vi "pump rpm all tubing.vi"(0 "Pump":T1 {"0 to 1" format="%.2f"; "flow rate" format="%.2f"}, 1 "pump ID":u8) -> (2 "pump U8":u8, 3 "pump speed (rpm)":dbl format="%.2f", 4 "command chars":string[](array[string]), 5 "in range":bool)   [LabVIEW 2012]
uses:
  Peristaltic/Pump w direction.ctl
  mini peristaltic pump.ctl
  Pump Direction.ctl
  3-stop colors and numbers.ctl
  calibration commands.ctl
panel:
  out "x+y":dbl
  in  "mL per rev":sgl[](array[numeric])=[0.001518497, 0.003209591, 0.005497798, 0.012406906, 0.016451517, 0.021816157, 0.026944764, 0.03351825, 0.04617598, 0.061704744, 0.069453366, 0.0789204, 0.088816434, 0.09612975, 0.10822253, 0.12075485, 0.14027181, 0.15709075, 0.17954482, 0.19715126, 0.2149444, 0.252498, 0.29306096, 0.3351765, 0.37380016, 0.42250744, 0.06, 0.21, 1.7, 0.8, 2.8, 3.8] format="%.7f"
  in  "IDs":sgl[](array[numeric])=[0.13, 0.19, 0.25, 0.38, 0.44, 0.51, 0.57, 0.64, 0.76, 0.89, 0.95, 1.02, 1.09, 1.14, 1.22, 1.3, 1.42, 1.52, 1.65, 1.75, 1.85, 2.06, 2.29, 2.54, 2.79, 3.17, 0.79375, 1.5875, 4.8, 3.175, 6.35, 7.9375] format="%.3f"
  # "orange-black\norange-red\norange-blue\norange-green\ngreen-yellow\norange-yellow\nwhite-yellow\norange-white\nblack-black\norange-orange\nwhite-black\nwhite-white\nwhite-red\nred-red\nred-grey\ngrey-grey\nyellow-yellow\nyellow-blue\nblue-blue\nblue-green\ngreen-green\npurple-purple\npurple-black\npurple-orange\npurple-white\nblack-white\n13\n14\n15\n16\n17\n18"
  # "13"
  # "14"
  # "15"
  # "16"
  # "17"
  # "18"
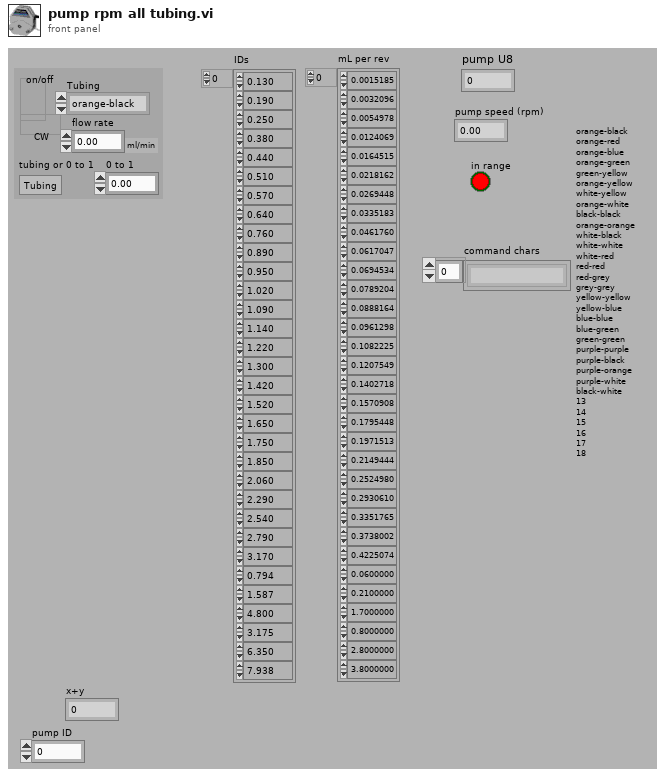
[diagram p1: front panel]
types:
  T1 = typedef "Pump w direction.ctl" = cluster{"on/off":T2, "Direction":T3, "flow rate":dbl[unit], "Tubing":T4, "tubing or 0 to 1":bool, "0 to 1":dbl}
  T2 = typedef "mini peristaltic pump.ctl" = bool
  T3 = typedef "Pump Direction.ctl" = bool
  T4 = typedef "3-stop colors and numbers.ctl" = enum16{"orange-black", "orange-red", "orange-blue", "orange-green", "green-yellow", "orange-yellow", "white-yellow", "orange-white", "black-black", "orange-orange", "white-black", "white-white", "white-red", "red-red", "red-grey", "grey-grey", "yellow-yellow", "yellow-blue", "blue-blue", "blue-green", "green-green", "purple-purple", "purple-black", "purple-orange", "purple-white", "black-white", "13", "14", "15", "16", "17", "18"}
  T5 = typedef "calibration commands.ctl" = enum16{"Get ini Path", "Save default values", "Save new calibration", "Read calibration", "Apply calibration", "Read STAMP mb", "Write STAMP mb"}
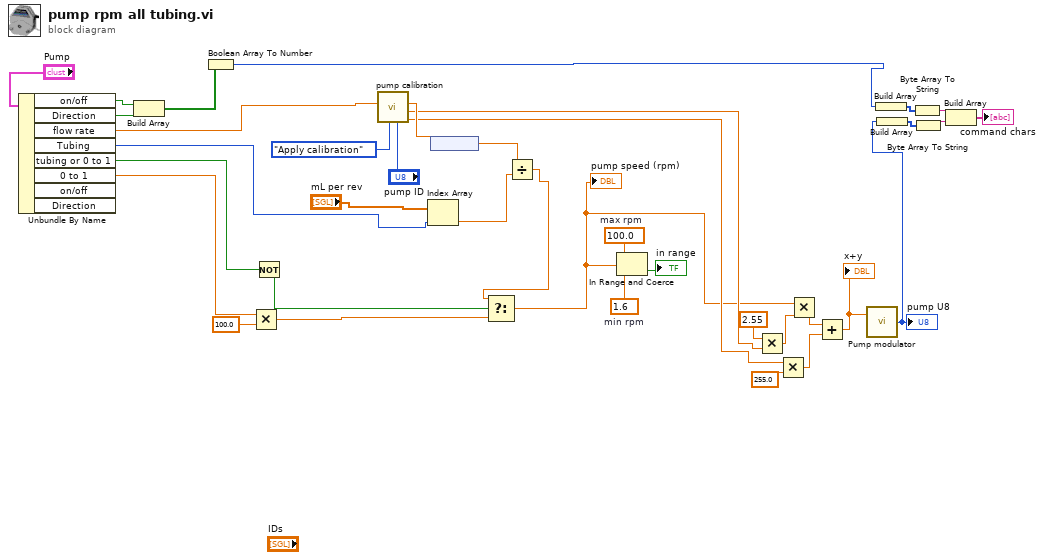
[diagram p0: block diagram]
diagram:
  w34 = 1.6  # min rpm
  w35 = 100.0  # max rpm
  n1 = Unbundle By Name("Pump") -> ("on/off"=w10:T2, "Direction"=w9:T3, "flow rate"=w29:dbl[unit], "Tubing"=w20:T4, "tubing or 0 to 1"=w19:bool, "0 to 1"=w18:dbl)  [unwired: 2 out]
  n2 = Build Array(w10, w9) -> (w11:T3[])
  n3 = Boolean Array To Number(Boolean array=w11) -> (number=w8:u32)
  n4 = Multiply(x=w18, y=100.0) -> (x*y=w15:dbl)
  n5 = Not(x=w19) -> (.not. x?=w13:bool)
  n6 = call "pump calibration.vi"("pump ID"="pump ID", "pump cal command"=calibration_commands."Apply calibration", "flow rate"=w29) -> ("STAMP intercept out"=w22:dbl, "STAMP slope out"=w23:dbl, "modified flow rate"=w32:dbl[unit])  [unwired: 5 in, 1 out]
  n7 = Index Array(array="mL per rev", index=w20) -> (element=w31:sgl)
  n8 = node(w32) -> (w36:dbl)
  n9 = Divide(x=w36, y=w31) -> (x/y=w16:dbl)
  n10 = Select(t=w16, s=w13, f=w15) -> (s? t:f=w17:dbl)
  "pump speed (rpm)" <- w17
  n11 = In Range and Coerce(upper limit=w35, x=w17, lower limit=w34) -> (In Range?=→"in range":bool)  [unwired: 1 out]
  n12 = Multiply(x=2.55, y=w23) -> (x*y=w26:dbl)
  n13 = Multiply(x=w22, y=255.0) -> (x*y=w27:dbl)
  n14 = Multiply(x=w17, y=w26) -> (x*y=w28:dbl)
  n15 = Add(x=w28, y=w27) -> (x+y=w25:dbl)
  "x+y" <- w25
  n16 = call "Pump modulator.vi"("y U8 in"=w25) -> ("y U8 modulated"=w3:u8)  [unwired: 1 in]
  "pump U8" <- w3
  n17 = Build Array(w8) -> (w7:u32[])
  n18 = Build Array(w3) -> (w5:u8[])
  n19 = Byte Array To String(unsigned byte array=w7) -> (string=w6:string)
  n20 = Byte Array To String(unsigned byte array=w5) -> (string=w4:string)
  n21 = Build Array(w6, w4) -> (→"command chars":string[])
